vi "Get Capacitance.vi"(8 "error in (no error)":errorcluster, 9 "Channel":i32, 11 "Instrument.CBridge in":refnum<class "Instrument.CBridge.lvclass">) -> (0 "error out":errorcluster, 2 "Capacitance (pF)":dbl, 3 "Instrument.CBridge out":refnum<class "Instrument.CBridge.lvclass">)   [LabVIEW 2019, in "Instrument.CBridge.lvclass"]
uses:
  Instrument.CBridge.lvclass
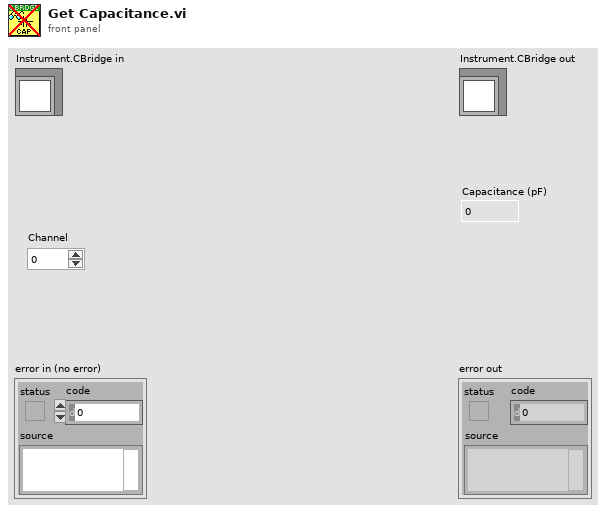
[diagram p1: front panel]
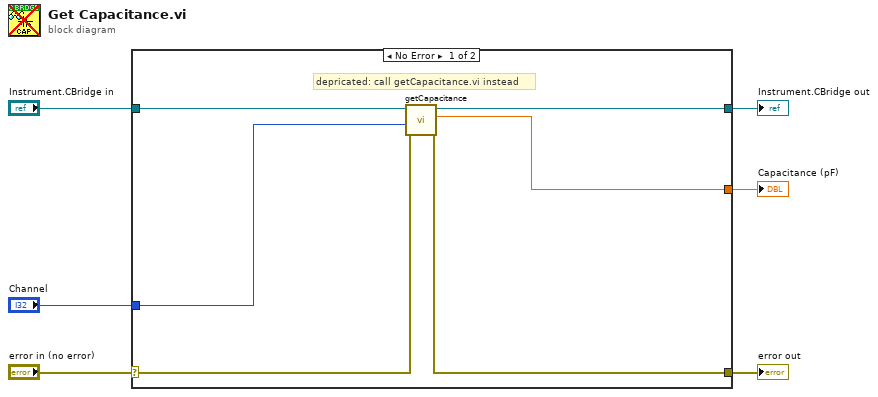
[diagram p0: block diagram]
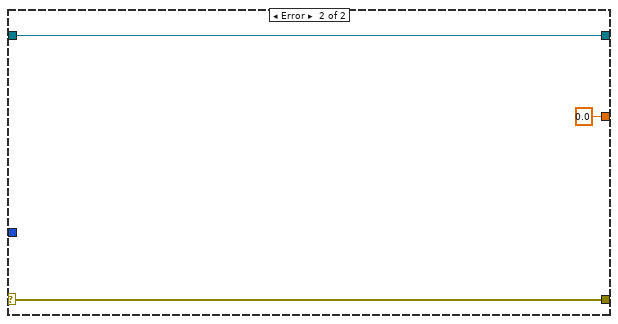
[diagram p2: hidden frame]
diagram:
  n1 = case shown="No Error" "error in (no error)" {
    selector: "error in (no error)" -> [w12 w15]
    tunnel: [w7 w15] -> w5
    tunnel: [w9 w14] -> w3
    tunnel: "Instrument.CBridge in" -> [w8 w14]
    tunnel: "Channel" -> [w11 _]
    tunnel: [w10 0.0 ("Capacitance (pF)")] -> w1
    frame No Error {
      # "depricated: call getCapacitance.vi instead"
      n2 = call-dynamic "getCapacitance.vi"("error in (no error)"=w12, "Channel"=w11, "Instrument.CBridge in"=w8) -> ("error out"=w7:errorcluster, "Capacitance (pF)"=w10:dbl, "Instrument.CBridge out"=w9:refnum<class "Instrument.CBridge.lvclass">)  [unwired: 6 in]
    }
    frame Error {
    }
  }
  "error out" <- w5
  "Instrument.CBridge out" <- w3
  "Capacitance (pF)" <- w1
